vi "practica113b.vi"() -> ()   [LabVIEW 2013]
uses:
  <vilib>/Native 3D Graph/xcontrol/3DPC_SurfacePlot.xctl
panel:
  in  "S3":i32
  in  "eje z":dbl
  out "3D Graph":refnum<class "Base Datatype.lvclass">[](xcontrol)
  out "S2 x":dbl
  out "S2 y":dbl
  out "S1 x":dbl
  out "S1 y":dbl
  in  "S2":i32
  in  "S1":i32
  in  "stop":bool
  in  "S2":dbl(knob) scale=-175.0..175.0
  in  "S1":dbl(knob) scale=0.0..360.0
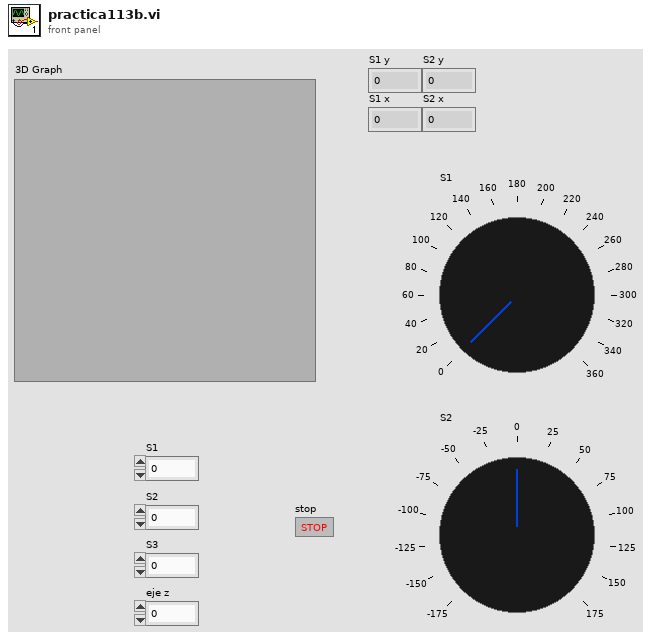
[diagram p1: front panel]
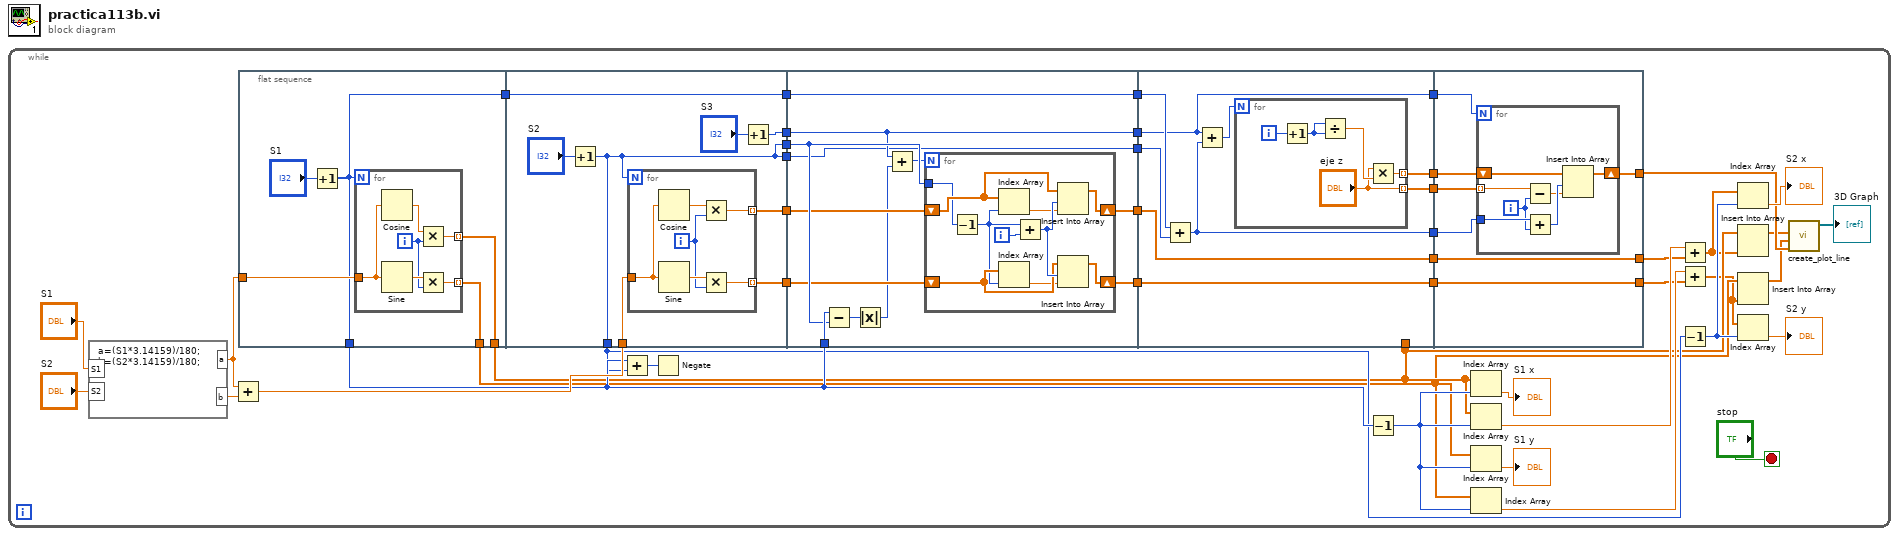
[diagram p0: block diagram]
diagram:
  n1 = while {
    stop <- "stop" stop-if-true
    n2 = formula code="a=(S1*3.14159)/180;\nb=(S2*3.14159)/180;"("S1"="S1", "S2"="S2") -> ("b"=w41:dbl, "a"=w40:dbl)
    n3 = Add(x=w40, y=w41) -> (x+y=w39:dbl)
    n4 = flat-sequence {
      tunnel: w40 -> [w50]
      tunnel: [w46] -> w28
      tunnel: [w48] -> w17
      tunnel: [w47] -> w19
      tunnel: [w46] -> w5
      tunnel: w39 -> [w63]
      tunnel: [w62] -> w37
      tunnel: [w61] -> w36
      tunnel: [w58] -> w35
      tunnel: [w58] -> w27
      tunnel: [w59] -> w10
      tunnel: [w58] -> w7
      tunnel: w5 -> [w57]
      tunnel: [w57] -> w4
      tunnel: w37 -> [w77]
      tunnel: w36 -> [w78]
      tunnel: w28 -> [w82]
      tunnel: w35 -> [w81]
      tunnel: [w79] -> w23
      tunnel: [w80] -> w22
      tunnel: w10 -> [w75]
      tunnel: [w75] -> w9
      tunnel: w7 -> [w74]
      tunnel: [w74] -> w6
      tunnel: w4 -> [w73]
      tunnel: [w73] -> w3
      tunnel: w23 -> [w100]
      tunnel: w22 -> [w101]
      tunnel: w19 -> [_]
      tunnel: [w100] -> w13
      tunnel: [w101] -> w12
      tunnel: [w99] -> w11
      tunnel: w9 -> [w95]
      tunnel: [w95] -> w8
      tunnel: w6 -> [w98]
      tunnel: w3 -> [w97]
      tunnel: [w96] -> w2
      tunnel: [w93] -> w1
      tunnel: [w108] -> w20
      tunnel: [w112] -> w32
      tunnel: [w113] -> w21
      tunnel: w13 -> [w113]
      tunnel: w12 -> [w112]
      tunnel: w11 -> [w109]
      tunnel: w8 -> [w111]
      tunnel: w2 -> [w107]
      tunnel: w1 -> [w110]
      frame #0 {
        n5 = Increment(x="S1") -> (x+1=w46:i32)
        n6 = for {
          N: w46 -> [_]
          tunnel: w50 -> [w52]
          tunnel: [w54] -> w48 mode=indexing
          tunnel: [w53] -> w47 mode=indexing
          i -> [w51]
          n7 = Cosine(x=w52) -> (cos(x)=w56:dbl)
          n8 = Sine(x=w52) -> (sin(x)=w55:dbl)
          n9 = Multiply(x=w56, y=w51) -> (x*y=w53:dbl)
          n10 = Multiply(x=w55, y=w51) -> (x*y=w54:dbl)
        }
      }
      frame #1 {
        n11 = Increment(x="S2") -> (x+1=w58:i32)
        n12 = for {
          N: w58 -> [_]
          tunnel: w63 -> [w66]
          tunnel: [w68] -> w61 mode=indexing
          tunnel: [w67] -> w62 mode=indexing
          i -> [w65]
          n13 = Cosine(x=w66) -> (cos(x)=w70:dbl)
          n14 = Sine(x=w66) -> (sin(x)=w69:dbl)
          n15 = Multiply(x=w70, y=w65) -> (x*y=w67:dbl)
          n16 = Multiply(x=w69, y=w65) -> (x*y=w68:dbl)
        }
        n17 = Increment(x="S3") -> (x+1=w59:i32)
      }
      frame #2 {
        n18 = Subtract(x=w82, y=w81) -> (x-y=w72:i32)
        n19 = Absolute Value(x=w72) -> (abs(x)=w71:i32)
        n20 = Add(x=w75, y=w71) -> (x+y=w76:i32)
        n21 = for {
          N: w76 -> [_]
          tunnel: w81 -> [w84]
          shift-right: [w88] -> w80
          shift-left: w78 -> [w90]
          shift-right: [w85] -> w79
          shift-left: w77 -> [w87]
          i -> [w92]
          n22 = Decrement(x=w84) -> (x-1=w83:i32)
          n23 = Index Array(array=w87, index=w83) -> (element=w86:dbl)
          n24 = Index Array(array=w90, index=w83) -> (element=w89:dbl)
          n25 = Add(x=w83, y=w92) -> (x+y=w91:i32)
          n26 = Insert Into Array(array=w87, index=w91, new element=w86) -> (w85:dbl[])
          n27 = Insert Into Array(array=w90, index=w91, new element=w89) -> (w88:dbl[])
        }
      }
      frame #3 {
        n28 = Add(x=w97, y=w98) -> (x+y=w93:i32)
        n29 = Add(x=w95, y=w93) -> (x+y=w94:i32)
        n30 = for {
          N: w94 -> [_]
          tunnel: [w105] -> w99 mode=indexing
          tunnel: ["eje z"] -> w96 mode=indexing
          i -> [w104]
          n31 = Increment(x=w104) -> (x+1=w103:i32)
          n32 = Divide(x=w103, y=w103) -> (x/y=w106:dbl)
          n33 = Multiply(x="eje z", y=w106) -> (x*y=w105:dbl)
        }
      }
      frame #4 {
        n34 = for {
          N: w111 -> [_]
          tunnel: w110 -> [w120]
          shift-right: [w115] -> w108
          shift-left: w109 -> [w118]
          tunnel: w107 -> [w117] mode=indexing
          i -> [w114]
          n35 = Subtract(x=w117, y=w114) -> (x-y=w116:dbl)
          n36 = Add(x=w120, y=w114) -> (x+y=w119:i32)
          n37 = Insert Into Array(array=w118, index=w119, new element=w116) -> (w115:dbl[])
        }
      }
    }
    n38 = Add(x=w28, y=w27) -> (x+y=w26:i32)
    n39 = Negate(x=w26) -> ()  [unwired: 1 out]
    n40 = Decrement(x=w28) -> (x-1=w24:i32)
    n41 = Index Array(array=w19, index=w24) -> (element=→"S1 x":dbl)
    n42 = Index Array(array=w19, index=w24) -> (element=w42:dbl)
    n43 = Index Array(array=w17, index=w24) -> (element=→"S1 y":dbl)
    n44 = Index Array(array=w17, index=w24) -> (element=w38:dbl)
    n45 = Add(x=w42, y=w21) -> (x+y=w18:dbl[])
    n46 = Add(x=w38, y=w32) -> (x+y=w16:dbl[])
    n47 = Decrement(x=w27) -> (x-1=w29:i32)
    n48 = Index Array(array=w18, index=w29) -> (element=→"S2 x":dbl)
    n49 = Insert Into Array(array=w19, new element=w18) -> (w15:dbl[])  [unwired: 1 in]
    n50 = Insert Into Array(array=w17, new element=w16) -> (w14:dbl[])  [unwired: 1 in]
    n51 = Index Array(array=w16, index=w29) -> (element=→"S2 y":dbl)
    n52 = call <vilib>:"create_plot_line.vi"("z vector"=w20, "y vector"=w14, "x vector"=w15) -> ("plots out"=→"3D Graph":refnum<class "Base Datatype.lvclass">[])  [unwired: 2 in, 6 out]
  }
